vi "Decorate.vi"(10 "Queue":refnum<class "Queue.lvclass">, 11 "qqqqq in":refnum<class "qqqqq.lvclass">) -> (3 "qqqqq out":refnum<class "qqqqq.lvclass">)   [LabVIEW 2021, in "jettl Tools.lvlib" / "qqqqq.lvlib" / "qqqqq.lvclass"]
uses:
  qqqqq.lvclass
  jettl/Queue/Queue.lvclass
  qqqqq.lvclass/qqqqq.ctl
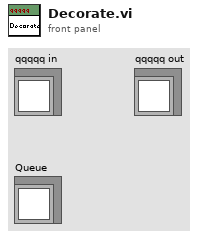
[diagram p1: front panel]
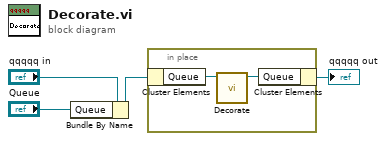
[diagram p0: block diagram]
diagram:
  n1 = Bundle By Name(cluster="qqqqq in", "Queue"="Queue") -> (w2:refnum<class "qqqqq.lvclass">)
  n2 = in-place {
    n3 = in-place-cluster #1(w2) -> ("Queue"=w6:refnum<class "Queue.lvclass">)
    n4 = call-dynamic "Decorate.vi"("Queue in"=w6) -> ("Queue out"=w5:refnum<class "Queue.lvclass">)  [unwired: 10 in]
    n5 = in-place-cluster #1("Queue"=w5) -> (→"qqqqq out":refnum<class "qqqqq.lvclass">)
  }
